vi "Get CITI Packages (Package Name).vi"(8 "error in (no error)":errorcluster, 10 "Package Name":string, 11 "CITI reference in":refnum<k24>) -> (0 "error out":errorcluster, 2 "CITI Package":T1, 3 "CITI reference out":refnum<k24>)   [LabVIEW 2023, in "NI_HFNetworkAnalysis.lvlib"]
doc: "Retrieve the CITI package in memory with the specified package name for the referenced CITI file."
uses:
  NI_HFNetworkAnalysis.lvlib
  C:/srd-semi-rfcal-software/AuxTools/STSRFFixtureCharactUtility/Source/Code Modules/Fixture/Dependencies/HFNetworkAnalysis/Support Files/NACE.Utils.Data.dll
  Support Files/NACE.Utils.Data.dll
  Controls/CITI Package.ctl
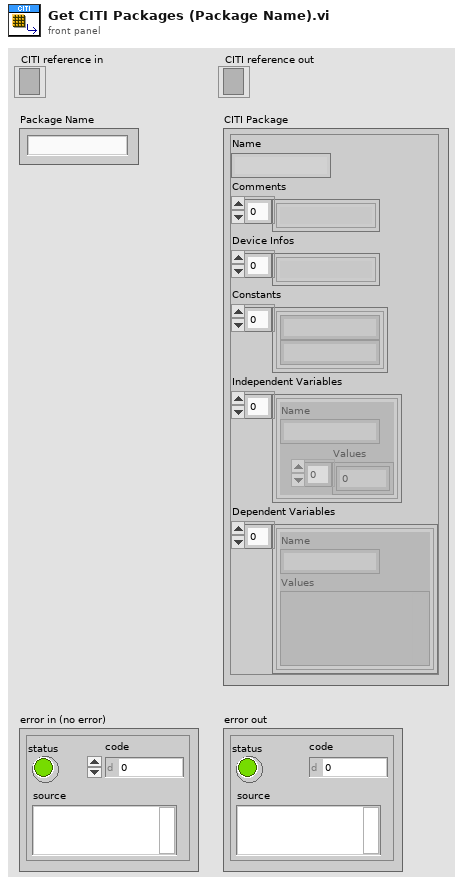
[diagram p1: front panel]
types:
  T1 = typedef "NI_HFNetworkAnalysis.lvlib/CITI Package.ctl" = cluster{"Name":string, "Comments":string[], "Device Infos":string[], "Constants":cluster{"Name":string, "Value":string}[], "Independent Variables":cluster{"Name":string, "Values":dbl[]}[], "Dependent Variables":cluster{"Name":string, "Values":variant}[]}
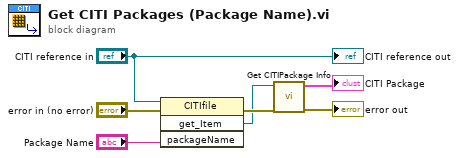
[diagram p0: block diagram]
diagram:
  n1 = invoke class="CITIfile" method="get_Item"(reference="CITI reference in", error in="error in (no error)", "packageName"="Package Name") -> (error out=w6:errorcluster, "get_Item"=w2:refnum<k24>)  [unwired: 1 in, 2 out]
  n2 = call "Get CITIPackage Info.vi"("error in (no error)"=w6, "CITI Package Refnum in"=w2) -> ("error out"=→"error out":errorcluster, "CITI Package"=→"CITI Package":T1)  [unwired: 8 in]
  "CITI reference out" <- "CITI reference in"
